vi "GammaGovernorHost.vi"() -> ()   [LabVIEW 2019]
uses:
  <vilib>/userDefined/High Color/nirio_resource_hc.ctl
  <vilib>/Analysis/2dsp.llb/Decimate (single shot, DBL).vi
  <vilib>/FPGAPlugInAG/USB-7845R/niLvFpga_Open_USB-7845R.vi
  <vilib>/rvi/interface/common/dynamic/niFpgaDynamicAddResources.vi
  <vilib>/FPGAPlugInAG/Dynamic/niLvFpga_Download_Dynamic.vi
  <vilib>/FPGAPlugInAG/Dynamic/niLvFpga_Reset_Dynamic.vi
  <vilib>/FPGAPlugInAG/Dynamic/niLvFpga_Run_Dynamic.vi
  <vilib>/Utility/error.llb/Error Cluster From Error Code.vi
  <vilib>/rvi/errors/niLvFpgaAdjustHostInterfaceError.vi
  <vilib>/express/express analysis/Spectral/Block/exnSpectralBlock spectral measurements PSD poly.vi
  <vilib>/express/express analysis/Spectral/Block/exnSpectralBlock spectral measurements PSD WFM.vi
  <vilib>/FPGAPlugInAG/Dynamic/niLvFpga_Close_Dynamic.vi
  <vilib>/rvi/interface/nirviOpenFPGA/nirviOpenFPGA.xnode
  FPGA Bitfiles/gammagovernor_FPGATarget_GammaGovernorTar_lSydMm8stKU.lvbitx
  Target/GammaGovernorTarget.vi
  <vilib>/rvi/interface/nirviMethod/nirviMethod.xnode
  <vilib>/express/express analysis/Spectral/XNode/ExpressSpectralMeasurementsBlockNode.xnode
  <vilib>/rvi/interface/nirviCloseFPGA/nirviCloseFPGA.xnode
  <vilib>/Analysis/NI_AALPro.lvlib
  <vilib>/FPGAPlugInAG/Dynamic/niLvFpga_ReadFifo_Dynamic.vi
  <vilib>/rvi/errors/niLvFpgaMergeErrorWithErrorCode.vi
panel:
  in  "Start":bool
  in  "Stop":bool
  in  "FPGA Target Device":T1
  out "Spectrogram Left":dbl[][](graph)
  out "Spectrogram Right":dbl[][](graph)
  out "Monitoring signals":T2(graph)
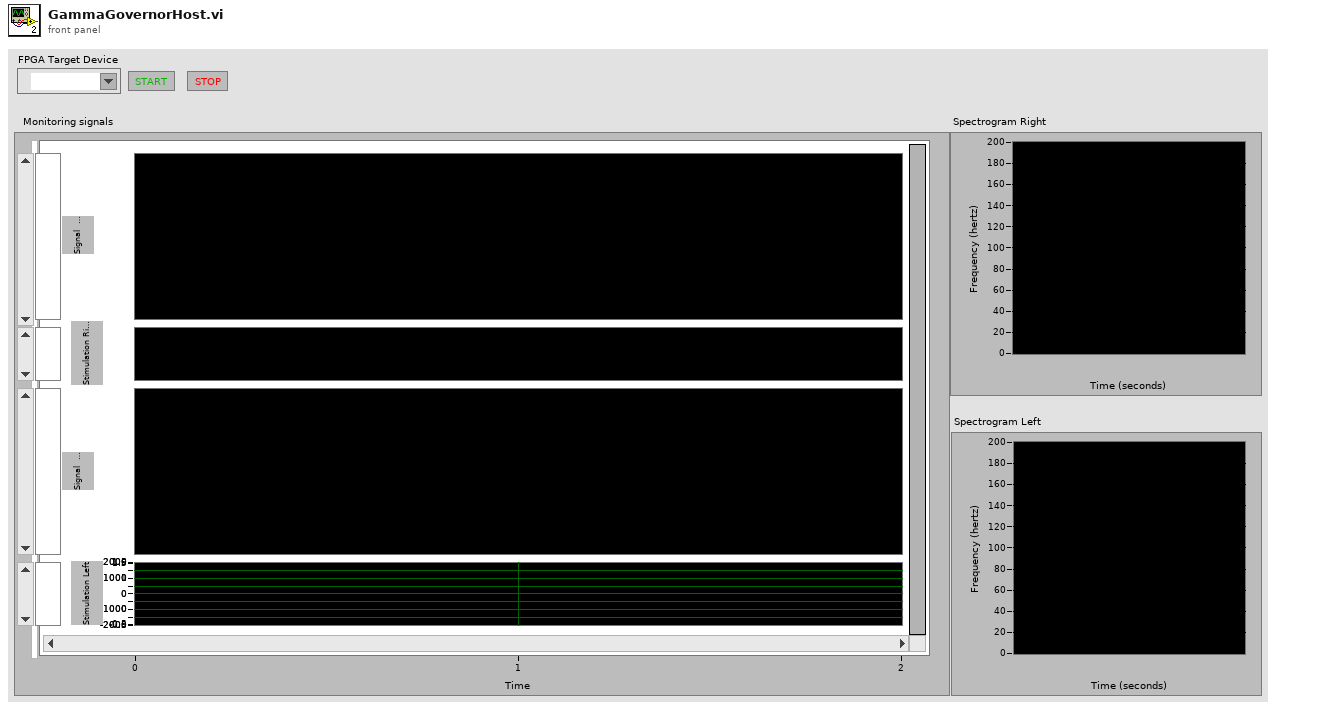
[diagram p1: front panel]
types:
  T1 = typedef "nirio_resource_hc.ctl" = tag
  T2 = cluster{waveform(u8), waveform(dbl), waveform(u8), waveform(dbl)}
  T3 = cluster{"averaging mode":u16, "weighting mode":u16, "number of averages":u32}
  T4 = cluster{"dB On (F)":bool, "unwrap phase (F)":bool, "convert to degree (F)":bool}
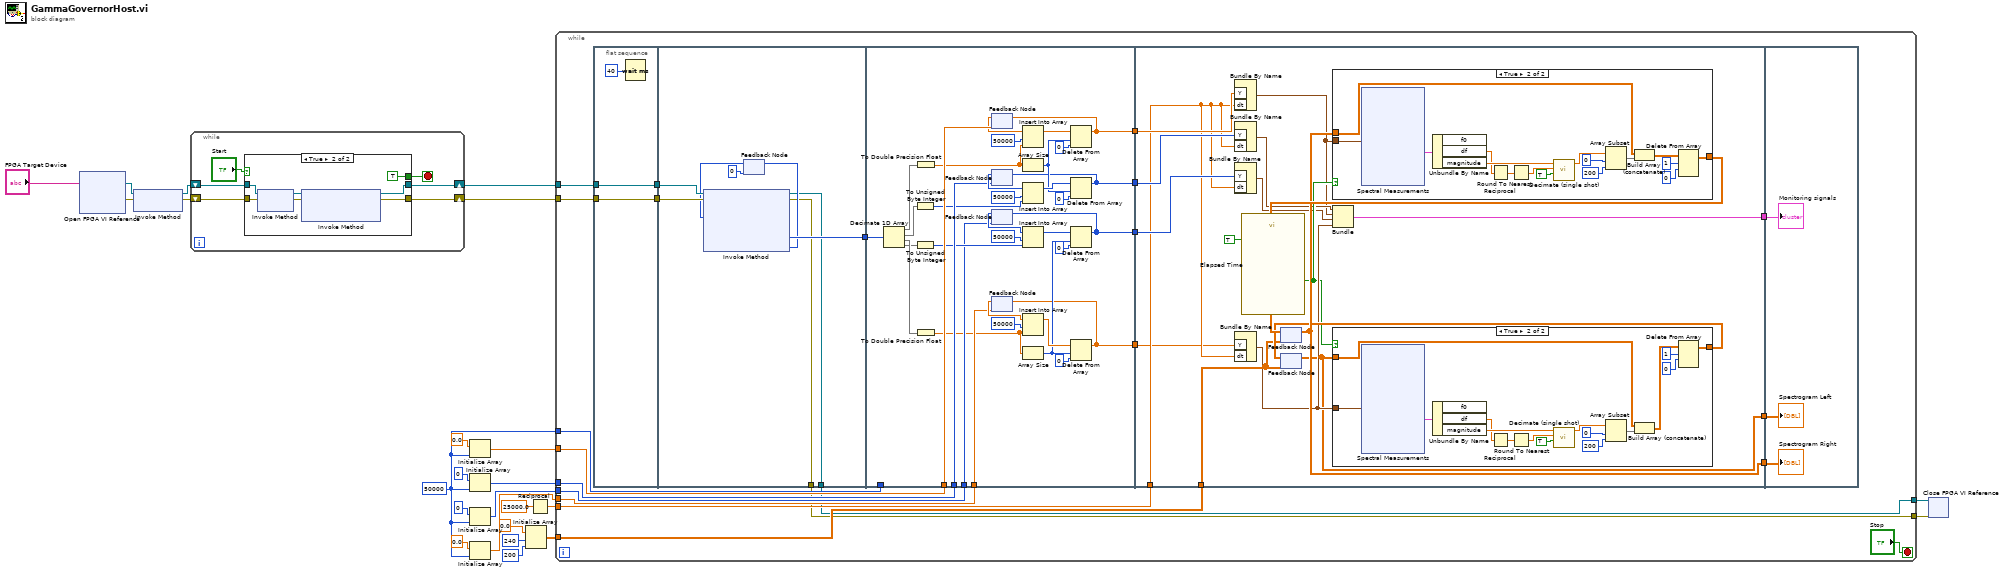
[diagram p0: block diagram]
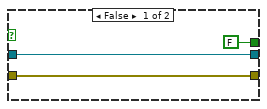
[diagram p2: hidden frame]
diagram:
  w12 = 50000 ("dimension size")
  n1 = xnode "Open FPGA VI Reference"("resource name"="FPGA Target Device") -> ("FPGA VI Reference Out"=w6:refnum<k20>, "error out"=w5:errorcluster)  [unwired: 1 in]
  n2 = xnode "Invoke Method"("FPGA VI Reference In"=w6, "error in"=w5) -> ("FPGA VI Reference Out"=w2:refnum<k20>, "error out"=w1:errorcluster)
  n3 = while {
    shift-right: [w29] -> w23
    shift-left: w2 -> [w28]
    shift-right: [w30] -> w24
    shift-left: w1 -> [w27]
    stop <- w25 stop-if-true
    n4 = case shown="True" "Start" {
      tunnel: [w32 w40] -> w30
      tunnel: [w33 w39] -> w29
      tunnel: w28 -> [w33 w37]
      tunnel: w27 -> [w32 w36]
      tunnel: [FALSE TRUE] -> w25
      frame False {
      }
      frame True {
        n5 = xnode "Invoke Method"("FPGA VI Reference In"=w37, "error in"=w36) -> ("FPGA VI Reference Out"=w35:refnum<k20>, "error out"=w34:errorcluster)
        n6 = xnode "Invoke Method"("FPGA VI Reference In"=w35, "error in"=w34) -> ("FPGA VI Reference Out"=w39:refnum<k20>, "error out"=w40:errorcluster)  [unwired: 1 in]
      }
    }
  }
  n7 = Initialize Array(0.0 ("element"), w12) -> (w21:dbl[])
  n8 = Initialize Array(u8 0 ("element"), w12) -> (w17:u8[])
  n9 = Initialize Array(u8 0 ("element"), w12) -> (w14:u8[])
  n10 = Initialize Array(0.0 ("element"), w12) -> (w13:dbl[])
  n11 = Initialize Array(0.0 ("element"), 240 ("dimension size"), 200 ("dimension size")) -> (w8:dbl[][])
  n12 = Reciprocal(x=25000.0) -> (1/x=w19:dbl)
  n13 = while {
    tunnel: w24 -> [w61]
    tunnel: w23 -> [w62]
    tunnel: w21 -> [w59]
    tunnel: w12 -> [w58]
    tunnel: w19 -> [w44]
    tunnel: w17 -> [w56]
    tunnel: w14 -> [w51]
    tunnel: w13 -> [w50]
    tunnel: w8 -> [w47]
    tunnel: [w42] -> w4
    tunnel: [w41] -> w3
    stop <- "Stop" stop-if-true
    n14 = flat-sequence {
      tunnel: w62 -> [w65]
      tunnel: w61 -> [w64]
      tunnel: [w65] -> w53
      tunnel: [w64] -> w52
      tunnel: [w73] -> w60
      tunnel: w53 -> [w72]
      tunnel: w52 -> [w71]
      tunnel: [w67] -> w42
      tunnel: [w66] -> w41
      tunnel: w60 -> [w108]
      tunnel: w59 -> [w107]
      tunnel: w58 -> [_]
      tunnel: [w102] -> w57
      tunnel: w56 -> [w97]
      tunnel: [w94] -> w55
      tunnel: w51 -> [w79]
      tunnel: w50 -> [w78]
      tunnel: [w77] -> w49
      tunnel: [w76] -> w48
      tunnel: w44 -> [w111]
      tunnel: w57 -> [w112]
      tunnel: w55 -> [w125]
      tunnel: [w124] -> w54
      tunnel: w49 -> [w123]
      tunnel: w48 -> [w110]
      tunnel: w47 -> [w118]
      tunnel: [w120] -> w46
      tunnel: [w115] -> w45
      tunnel: w54 -> [w182]
      tunnel: w46 -> [w181]
      tunnel: w45 -> [w180]
      frame #0 {
        n15 = Wait (ms)(milliseconds to wait=u32 40) -> ()  [unwired: 1 out]
      }
      frame #1 {
        n16 = feedback #1(u32 0 ("Elements Remaining")) -> (w69:u32)
        n17 = xnode "Invoke Method"("FPGA VI Reference In"=w72, "error in"=w71, "Number of Elements"=w69) -> ("FPGA VI Reference Out"=w67:refnum<k20>, "error out"=w66:errorcluster, "Data"=w73:i16[], "Elements Remaining"=w70:u32)  [unwired: 1 in]
        n18 = feedback-in #1(w70) -> ()
      }
      frame #2 {
        n19 = Decimate 1D Array(w108) -> (w93:i16[], w92:i16[], w81:i16[], w80:i16[])
        n20 = To Unsigned Byte Integer(number=w92) -> (unsigned 8bit integer=w95:u8[])
        n21 = To Unsigned Byte Integer(number=w80) -> (unsigned 8bit integer=w82:u8[])
        n22 = To Double Precision Float(number=w93) -> (double precision float=w75:dbl[])
        n23 = To Double Precision Float(number=w81) -> (double precision float=w74:dbl[])
        n24 = feedback #2(w107) -> (w106:dbl[])
        n25 = feedback #3(w97) -> (w101:u8[])
        n26 = feedback #4(w79) -> (w87:u8[])
        n27 = feedback #5(w78) -> (w91:dbl[])
        n28 = Insert Into Array(array=w106, index=50000, new element=w75) -> (w103:dbl[])
        n29 = Array Size(array=w75) -> (size(s)=w96:i32)
        n30 = Insert Into Array(array=w101, index=50000, new element=w95) -> (w98:u8[])
        n31 = Insert Into Array(array=w87, index=50000, new element=w82) -> (w84:u8[])
        n32 = Insert Into Array(array=w91, index=50000, new element=w74) -> (w88:dbl[])
        n33 = Array Size(array=w74) -> (size(s)=w83:i32)
        n34 = Delete From Array(array=w103, length=w96, index=0) -> (array with subset deleted=w102:dbl[])  [unwired: 1 out]
        n35 = feedback-in #2(w102) -> ()
        n36 = Delete From Array(array=w98, length=w96, index=0) -> (array with subset deleted=w94:u8[])  [unwired: 1 out]
        n37 = feedback-in #3(w94) -> ()
        n38 = Delete From Array(array=w84, length=w83, index=0) -> (array with subset deleted=w77:u8[])  [unwired: 1 out]
        n39 = feedback-in #4(w77) -> ()
        n40 = Delete From Array(array=w88, length=w83, index=0) -> (array with subset deleted=w76:dbl[])  [unwired: 1 out]
        n41 = feedback-in #5(w76) -> ()
      }
      frame #3 {
        n42 = Bundle By Name("Y"=w112, "dt"=w111) -> (w113:waveform(dbl))  [unwired: 1 in]
        n43 = Bundle By Name("Y"=w125, "dt"=w111) -> (w114:waveform(u8))  [unwired: 1 in]
        n44 = Bundle By Name("Y"=w123, "dt"=w111) -> (w109:waveform(u8))  [unwired: 1 in]
        n45 = Bundle By Name("Y"=w110, "dt"=w111) -> (w117:waveform(dbl))  [unwired: 1 in]
        n46 = call "Elapsed Time"("Auto Reset"=TRUE) -> ("Time has Elapsed"=w116:bool)  [unwired: 11 in, 7 out]
        n47 = feedback #6(w118) -> (w120:dbl[][])
        n48 = feedback #7(w118) -> (w115:dbl[][])
        n49 = case shown="True" w116 {
          tunnel: w113 -> [_ w160]
          tunnel: [w153 w155] -> w121
          tunnel: w120 -> [w153 w154]
          frame False {
          }
          frame True {
            n50 = xnode "Spectral Measurements"("Signals"=w160) -> ("PSD"=w161:cluster{"f0":dbl, "df":dbl, "magnitude":dbl[]})  [unwired: 2 in, 2 out]
            n51 = Unbundle By Name(w161) -> ("df"=w162:dbl, "magnitude"=w166:dbl[])  [unwired: 1 out]
            n52 = Reciprocal(x=w162) -> (1/x=w163:dbl)
            n53 = Round To Nearest(number=w163) -> (nearest integer value=w164:dbl)
            n54 = call-poly <vilib>:"Decimate (single shot).vi"("averaging"=TRUE, "decimating factor"=w164, "X"=w166) -> ("Decimated Array"=w167:dbl[])  [unwired: 7 in, 1 out]
            n55 = Array Subset(array=w167, index=0, length=200) -> (w159:dbl[])
            n56 = Build Array (concatenate)(w154, w159) -> (w158:dbl[][])
            n57 = Delete From Array(array=w158, length=1, index (row)=0) -> (array with subset deleted=w155:dbl[][])  [unwired: 1 in, 1 out]
          }
        }
        n58 = feedback-in #6(w121) -> ()
        n59 = Bundle(w114, w113, w109, w117) -> (w124:T2)  [unwired: 1 in]
        n60 = case shown="True" w116 {
          tunnel: [w126 w129] -> w119
          tunnel: w117 -> [_ w128]
          tunnel: w115 -> [w126 w127]
          frame False {
          }
          frame True {
            n61 = xnode "Spectral Measurements"("Signals"=w128) -> ("PSD"=w134:cluster{"f0":dbl, "df":dbl, "magnitude":dbl[]})  [unwired: 2 in, 2 out]
            n62 = Unbundle By Name(w134) -> ("df"=w135:dbl, "magnitude"=w139:dbl[])  [unwired: 1 out]
            n63 = Reciprocal(x=w135) -> (1/x=w136:dbl)
            n64 = Round To Nearest(number=w136) -> (nearest integer value=w137:dbl)
            n65 = call-poly <vilib>:"Decimate (single shot).vi"("averaging"=TRUE, "decimating factor"=w137, "X"=w139) -> ("Decimated Array"=w140:dbl[])  [unwired: 7 in, 1 out]
            n66 = Array Subset(array=w140, index=0, length=200) -> (w133:dbl[])
            n67 = Build Array (concatenate)(w127, w133) -> (w132:dbl[][])
            n68 = Delete From Array(array=w132, length=1, index (row)=0) -> (array with subset deleted=w129:dbl[][])  [unwired: 1 in, 1 out]
          }
        }
        n69 = feedback-in #7(w119) -> ()
      }
      frame #4 {
        "Monitoring signals" <- w182
        "Spectrogram Right" <- w181
        "Spectrogram Left" <- w180
      }
    }
  }
  n70 = xnode "Close FPGA VI Reference"("FPGA VI Reference In"=w4, "error in"=w3) -> ()  [unwired: 1 out]
